vi "Set MXN.vi"(8 "error in (no error)":errorcluster, 10 "MXN":bool, 11 "Soda Actors in":refnum<class "Soda Actors.lvclass">) -> (0 "error out":errorcluster, 3 "Soda Actors out":refnum<class "Soda Actors.lvclass">)   [LabVIEW 2020, in "Soda Actors.lvlib" / "Soda Actors.lvclass"]
uses:
  Soda Actors.lvclass
  Soda Actors.lvclass/Soda Actors.ctl
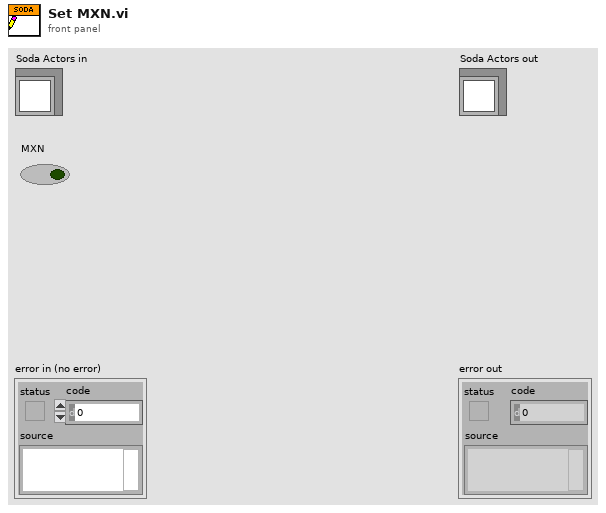
[diagram p1: front panel]
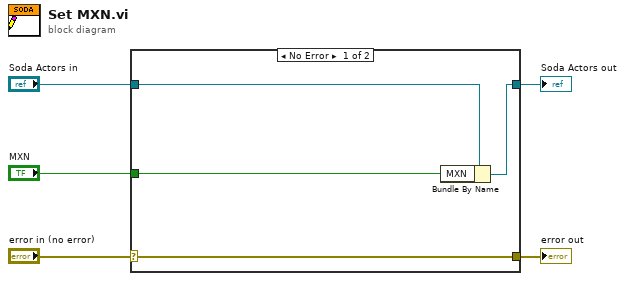
[diagram p0: block diagram]
diagram:
  n1 = case shown="No Error" "error in (no error)" {
    selector: "error in (no error)" -> [w9 w10]
    tunnel: [w9 w10] -> w4
    tunnel: [w7 w11] -> w2
    tunnel: "Soda Actors in" -> [w8 w11]
    tunnel: "MXN" -> [w6 _]
    frame No Error {
      n2 = Bundle By Name(cluster=w8, "MXN"=w6) -> (w7:refnum<class "Soda Actors.lvclass">)
    }
    frame Error {
    }
  }
  "error out" <- w4
  "Soda Actors out" <- w2
